vi "ROI grp-Case-Recover previous setup.vi"(11 "POI groups initial setup":T1 {"Groups setup out"."Group region specifier cluster"."Contours"."Type" items=["No Selection", "Point", "Line", "Rectangle", "Oval", "Polygon", "Freehand Region", "Annulus", "Unused2", "Unused3", "Broken Line", "Freehand Line", "Rotated Rectangle"]}) -> (0 "error out":errorcluster, 3 "Window close was cancelled":bool)   [LabVIEW 2017]
uses:
  Typedefs/ROI grp-Internal register.ctl
  ROI Selection Interface/ROI group info cluster.ctl
  Typedefs/Group sel cluster.ctl
  Experiment header interface/Typedefs/Save-Load-Save as-Load last enum.ctl
  Globals/gl_ROI grp window globals.vi
  Global variables/gl_Functional Imaging-Global variables.vi
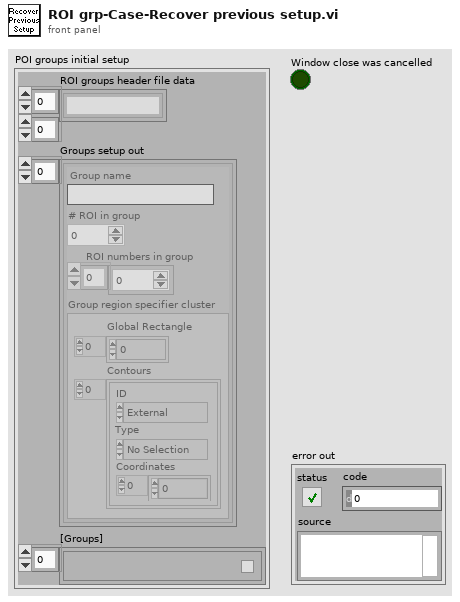
[diagram p1: front panel]
types:
  T1 = typedef "ROI grp-Internal register.ctl" = cluster{"ROI groups header file data":string[][], "Groups setup out":T2[], "[Groups]":T4[]}
  T2 = typedef "ROI group info cluster.ctl" = cluster{"Group name":string, "# ROI in group":i32, "ROI numbers in group":i32[], "Group region specifier cluster":T3}
  T3 = typedef "ROI Descriptor" = cluster{"Global Rectangle":i32[], "Contours":cluster{"ID":enum32{"External", "Internal"}, "Type":u32, "Coordinates":i32[]}[]}
  T4 = typedef "Group sel cluster.ctl" = cluster{"Group number":string, "Group Name":string, "Visibility":bool, "Highlight":bool}
  T5 = typedef "Save-Load-Save as-Load last enum.ctl" = enum16{"Save file", "Save file as", "Load file", "Load last file"}
  T6 = typedef "ROI grp-window ctrl refs.ctl" = cluster{"This VI":refnum<vi>, "Pane":refnum<vi>, "Table":refnum<vi>}
  T7 = typedef "Functional Imging UI Refs.ctl" = cluster{"Menu ref":refnum<k9>, "Image control":refnum<vi>, "VI ref":refnum<vi>, "XGrapher":refnum<vi>, "Smoothing":refnum<vi>, "POI Averaging":refnum<vi>, "Normalize":refnum<vi>, "POI data points in each trial":refnum<vi>, "Channel":refnum<vi>, "Experiment data folder path":refnum<vi>, "[ROI vis]":refnum<vi>, "[Groups] visbl":T8, "Group Name":refnum<vi>, "POI index":refnum<vi>, "Trial No.":refnum<vi>, "Intensity Zoom":refnum<vi>, "Trial Cursor Enabled":refnum<vi>, "Number of Trials (ind 1)":refnum<vi>, "Number of Trials (ind 2)":refnum<vi>, "MiniScans Available":refnum<vi>, "POI Available":refnum<vi>, "Defer graph updates":refnum<vi>, "Waveform selector":refnum<vi>, "#of selected POI":refnum<vi>, "#of selected MiniScans":refnum<vi>, "#of selected groups":refnum<vi>, "Max Z-Projection":refnum<vi>, "Z-Plane Selector":refnum<vi>, "Index of miniscan point to visualise":refnum<vi>, "ROI vis. mode":refnum<vi>, "Total # of points":refnum<vi>, "Index of group clicked on":refnum<vi>, "Pane 1":refnum<vi>, "Pane 2":refnum<vi>, "Pane 3":refnum<vi>, "Pane 4":refnum<vi>, "Pane 5":refnum<vi>, "Pane 6":refnum<vi>, "Deselect all ROI":refnum<vi>, "Deselect all groups":refnum<vi>}
  T8 = typedef "Groups array referecne.ctl" = refnum<vi>
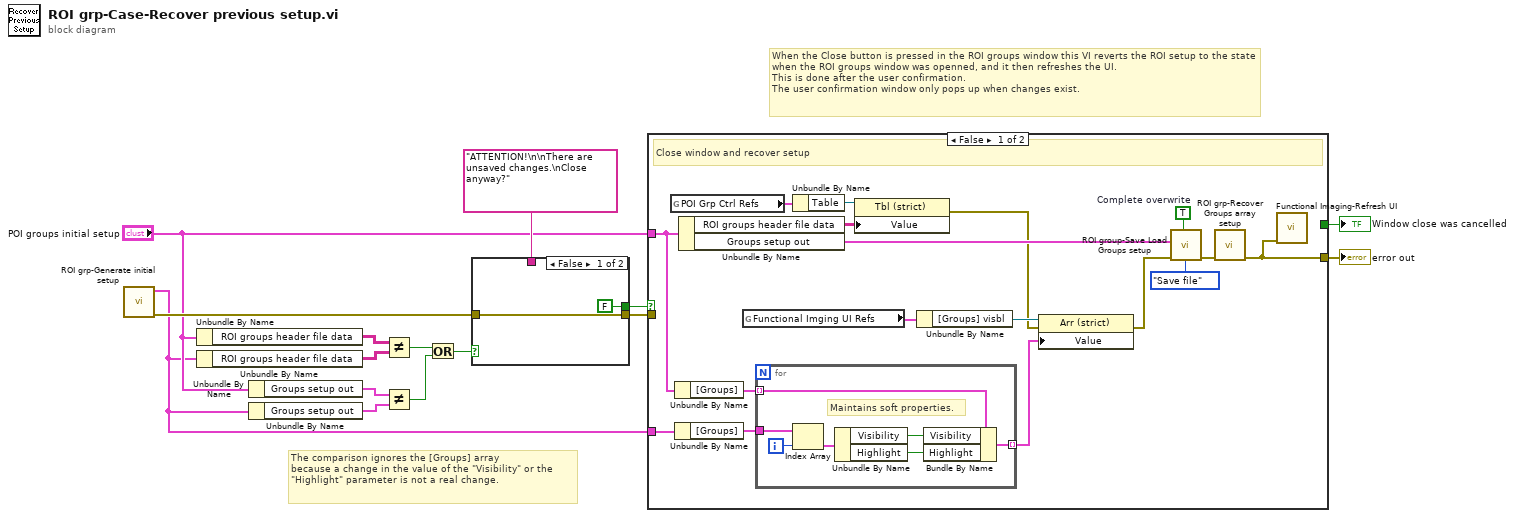
[diagram p0: block diagram]
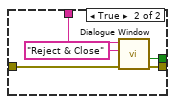
[diagram p2: hidden frame]
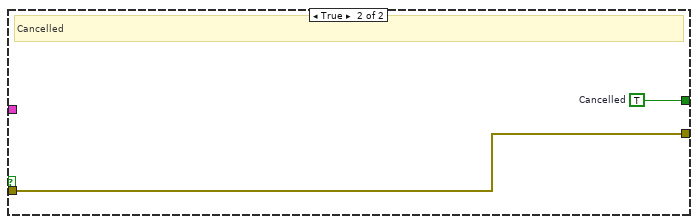
[diagram p3: hidden frame]
diagram:
  # "The comparison ignores the [Groups] array\nbecause a change in the value of the \"Visibility\" or the \"Highlight\" parameter is not a real change."
  # "When the Close button is pressed in the ROI groups window this VI reverts the ROI setup to the state when the ROI groups window was openned, and it then refreshes the UI.\nThis is done after the user confirmation.\nThe user confirmation window only pops up when changes exist."
  n1 = call "ROI grp-Generate initial setup.vi"() -> ("error out"=w12:errorcluster, "ROI groups new setup"=w1:T1)  [unwired: 10 in]
  n2 = Unbundle By Name("POI groups initial setup") -> ("ROI groups header file data"=w7:string[][])
  n3 = Unbundle By Name(w1) -> ("ROI groups header file data"=w6:string[][])
  n4 = Unbundle By Name("POI groups initial setup") -> ("Groups setup out"=w4:T2[])
  n5 = Unbundle By Name(w1) -> ("Groups setup out"=w5:T2[])
  n6 = Not Equal?(x=w7, y=w6) -> (x != y?=w3:bool)
  n7 = Not Equal?(x=w4, y=w5) -> (x != y?=w2:bool)
  n8 = Or(x=w3, y=w2) -> (x .or. y?=w8:bool)
  n9 = case shown="False" w8 {
    tunnel: "ATTENTION!\n\nThere are unsaved changes.\nClose anyway?" ("Message string") -> [_ w22]
    tunnel: [FALSE ("Cancelled (Left button pressed)") w20] -> w13
    tunnel: w12 -> [w17 w19]
    tunnel: [w17 w18] -> w11
    frame False {
    }
    frame True {
      n10 = call "Dialogue Window.vi"("error in (no error)"=w19, "Caption-Right button (OK)"="Reject & Close", "Message string"=w22) -> ("error out"=w18:errorcluster, "Cancelled (Left button pressed)"=w20:bool)  [unwired: 6 in, 1 out]
    }
  }
  n11 = case shown="False" w13 {
    tunnel: [w33 w48] -> w15
    tunnel: "POI groups initial setup" -> [w24 _]
    tunnel: w11 -> [_ w48]
    tunnel: [_ w47] -> w10
    tunnel: w1 -> [w26 _]
    frame False {
      w36 = TRUE  # Complete overwrite
      # "Close window and recover setup"
      n12 = global read "gl_ROI grp window globals.vi" "POI Grp Ctrl Refs"() -> (w37:T6)
      n13 = Unbundle By Name(w24) -> ("[Groups]"=w23:T4[])
      n14 = Unbundle By Name(w26) -> ("[Groups]"=w25:T4[])
      n15 = Unbundle By Name(w24) -> ("ROI groups header file data"=w39:string[][], "Groups setup out"=w30:T2[])
      n16 = global read "gl_Functional Imaging-Global variables.vi" "Functional Imging UI Refs"() -> (w32:T7)
      n17 = for {
        tunnel: w23 -> [w46] mode=indexing
        tunnel: [w45] -> w27 mode=indexing
        tunnel: w25 -> [w44]
        i -> [w43]
        # "Maintains soft properties."
        n18 = Index Array(array=w44, index=w43) -> (element=w42:T4)
        n19 = Unbundle By Name(w42) -> ("Visibility"=w41:bool, "Highlight"=w40:bool)
        n20 = Bundle By Name(cluster=w46, "Visibility"=w41, "Highlight"=w40) -> (w45:T4)
      }
      n21 = Unbundle By Name(w37) -> ("Table"=w38:refnum<vi>)
      n22 = property on="Property Node" class="Tbl (strict)"(reference=w38, "Value"=w39) -> (error out=w29:errorcluster)  [unwired: 1 in, 1 out]
      n23 = Unbundle By Name(w32) -> ("[Groups] visbl"=w31:T8)
      n24 = property on="Property Node" class="Arr (strict)"(reference=w31, error in=w29, "Value"=w27) -> (error out=w28:errorcluster)  [unwired: 1 out]
      n25 = call "ROI group-Save Load Groups setup.vi"("error in (no error)"=w28, "Function"=Save-Load-Save_as-Load_last_enum."Save file", "Groups setup to save"=w30, "Complete overwrite (F)"=w36) -> ("error out"=w34:errorcluster)  [unwired: 6 in, 1 out]
      n26 = call "ROI grp-Recover Groups array setup.vi"("error in (no error)"=w34) -> ("error out"=w33:errorcluster)  [unwired: 10 in]
      n27 = call "Functional Imaging-Refresh UI.vi"("error in (no error)"=w33) -> ()  [unwired: 11 in]
    }
    frame True {
      w47 = TRUE  # Cancelled
      # "Cancelled"
    }
  }
  "error out" <- w15
  "Window close was cancelled" <- w10
